vi "Close.vi"(8 "error in (no error)":errorcluster, 11 "Impersonate in":refnum<class "LogonUser.lvclass">) -> (0 "error out":errorcluster, 3 "Impersonate out":refnum<class "LogonUser.lvclass">)   [LabVIEW 2018, in "LogonUser.lvclass"]
doc: "©2019\nWiebe Walstra\nwww.carya.nl"
uses:
  LogonUser.lvclass
  LogonUser.lvclass/LogonUser.ctl
  kernel32.dll
  advapi32.dll
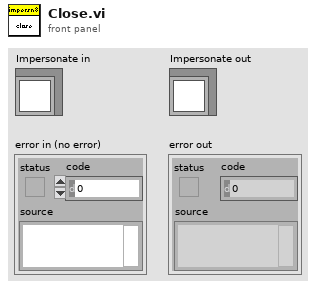
[diagram p1: front panel]
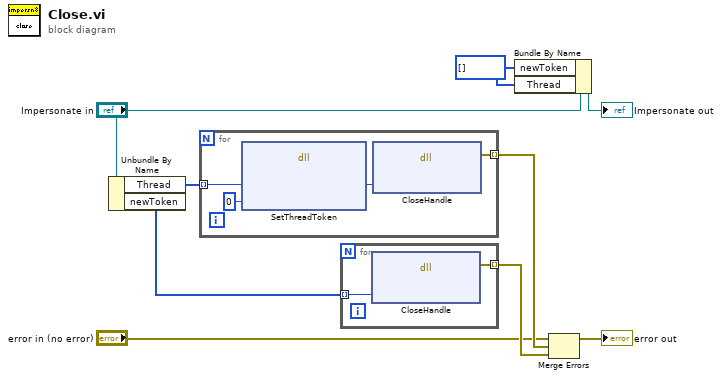
[diagram p0: block diagram]
diagram:
  w1 = i64[] [] ("newToken")
  n1 = Unbundle By Name("Impersonate in") -> ("Thread"=w6:i64[], "newToken"=w7:i64[])
  n2 = for {
    tunnel: w6 -> [w13] mode=indexing
    tunnel: [w12] -> w5 mode=indexing
    n3 = dll-call lib="Advapi32.dll" fn="SetThreadToken"("pThread"=w13, "newToken"=i64 0) -> ("pThread"=w10:i64)  [unwired: 5 in, 2 out]
    n4 = dll-call lib="kernel32.dll" fn="CloseHandle"("handle"=w10) -> (error out=w12:errorcluster)  [unwired: 5 in, 1 out]
  }
  n5 = for {
    tunnel: w7 -> [w15] mode=indexing
    tunnel: [w14] -> w4 mode=indexing
    n6 = dll-call lib="kernel32.dll" fn="CloseHandle"("handle"=w15) -> (error out=w14:errorcluster)  [unwired: 5 in, 1 out]
  }
  n7 = Bundle By Name(cluster="Impersonate in", "newToken"=w1, "Thread"=w1) -> (→"Impersonate out":refnum<class "LogonUser.lvclass">)
  n8 = Merge Errors("error in (no error)", w5, w4) -> (→"error out":errorcluster)
